vi "Report.vi"(6 "Printer Name":string, 8 "error in":errorcluster, 10 "Print/Preview":bool, 11 "Data In":T1) -> (0 "error out":errorcluster, 3 "Data Out":T1)   [LabVIEW 2025]
uses:
  <vilib>/Utility/NIReport.llb/NI_report.lvclass
  <vilib>/Utility/NIReport.llb/image depth.ctl
  <vilib>/Utility/NIReport.llb/NI_ReportGenerationCore.lvlib
  <vilib>/Utility/NIReport.llb/Report Type.ctl
  <vilib>/Utility/NIReport.llb/HTML Report Image Alignment.ctl
  <vilib>/Utility/NIReport.llb/Append Report Text (str wrap).vi
  <vilib>/printing/OpenHTMLReport.llb/Open HTML Report in Browser (Refnum).vi
  Controls/Tension_Output.ctl
  Controls/Nippel Turn Direction.ctl
  Controls/Runout Output.ctl
  Controls/Aditional Info.ctl
  Controls/Spork plot.ctl
  Controls/Spork type.ctl
  Controls/Spoke_stats.ctl
  Controls/Tension.ctl
  Controls/Runout.ctl
  Controls/Wheel_data.ctl
panel:
  out "Aditional Information":T10
  out "Spork Measured":i32[](array[numeric])
  out "Runout Measurement":T8[](array[typedef]) caption="Runout Value      Adjustment"
  out "Tencion Left":T6[](array[typedef]) caption="Tencion Left [kgf]    Pass?"
  out "Tencion Right":T6[](array[typedef]) caption="Tencion Right [kgf]   Pass?"
  out "Spokes Tension":cluster{dbl[], dbl[]}[](graph)
  out "Runout":T2[](graph)
  out "Wheel Visualation":cluster{dbl[], dbl[]}[](graph)
  # "Tension [kgf]"
  # "Pass?"
  # "Tension [kgf]"
  # "Pass?"
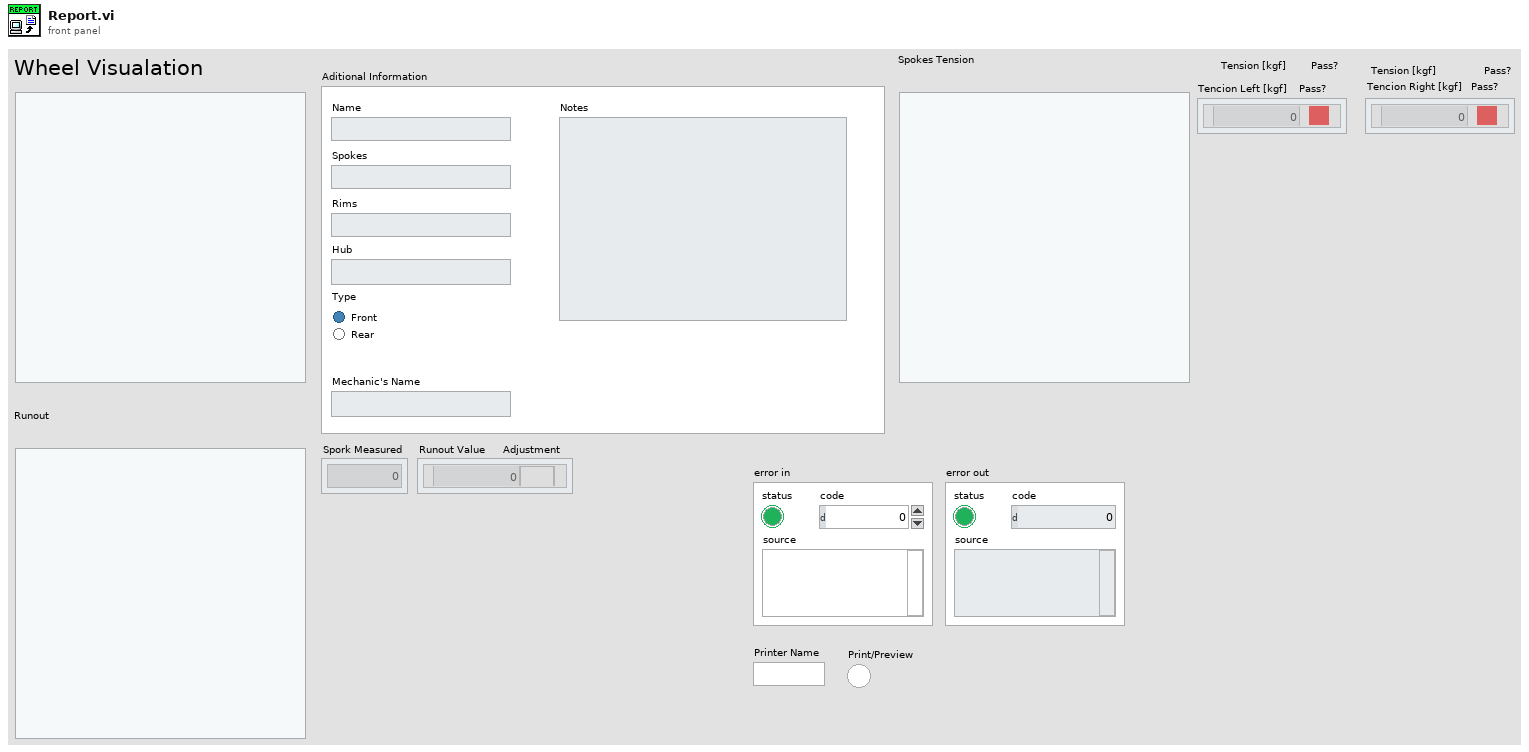
[diagram p1: front panel]
types:
  T1 = typedef "Wheel_data.ctl" = cluster{"Wheel Grapth":T2[], "Spokes":T3, "Tension":T5, "Runout":T7, "Avaliable Printers":string[], "Aditional Info":T10}
  T2 = typedef "Spork plot.ctl" = cluster{"X":dbl[], "Y":dbl[]}
  T3 = typedef "Spoke_stats.ctl" = cluster{"Spokes number":i32, "Spokes crosses":i32, "Spokes Type":T4}
  T4 = typedef "Spork type.ctl" = enum16{"Steel 1.4mm", "Steel 1.5mm", "Steel 1.6mm", "Steel 1.7mm", "Steel 1.8mm", "Steel 2mm", "Steel 2.3mm", "Steel 2.5mm", "Steel 2.6mm", "Aluminum 2.28mm", "Aluminum 2.54mm", "Aluminum 2.8mm", "Aluminum 3.3mm"}
  T5 = typedef "Tension.ctl" = cluster{"Spokes Tension Left":dbl[], "Tension Graph":T2[], "Average Left":dbl, "Variance":dbl, "Std Div Left":dbl, "Average Right":dbl, "Std Div Right":dbl, "Tension Output Left":T6[], "Tension Output Right":T6[], "Spokes Tension Right":dbl[]}
  T6 = typedef "Tension_Output.ctl" = cluster{"Tenction [kgf]":dbl, "Within Limit":bool}
  T7 = typedef "Runout.ctl" = cluster{"Runout Output":T8[], "Runout Graph":T2[], "Average":dbl, "Std Div":dbl, "Spoke Measured":i32[]}
  T8 = typedef "Runout Output.ctl" = cluster{"Value":dbl, "Nippel Direction":T9}
  T9 = typedef "Nippel Turn Direction.ctl" = u16
  T10 = typedef "Aditional Info.ctl" = cluster{"Name":string, "Rims":string, "Hub":string, "Notes":string, "Spokes":string, "Type":enum32{"Item 0", "Item 1"}, "Mechanic's Name":string}
  T11 = typedef "NI_ReportGenerationCore.lvlib/image depth.ctl" = u16
  T12 = typedef "NI_ReportGenerationCore.lvlib/HTML Report Image Alignment.ctl" = enum16{"(default)", "LEFT", "RIGHT", "TOP", "TEXTTOP", "MIDDLE", "ABSMIDDLE", "BASELINE", "BOTTOM", "ABSBOTTOM"}
  T13 = typedef "NI_ReportGenerationCore.lvlib/Report Type.ctl" = enum16{"HTML", "Word", "Excel"}
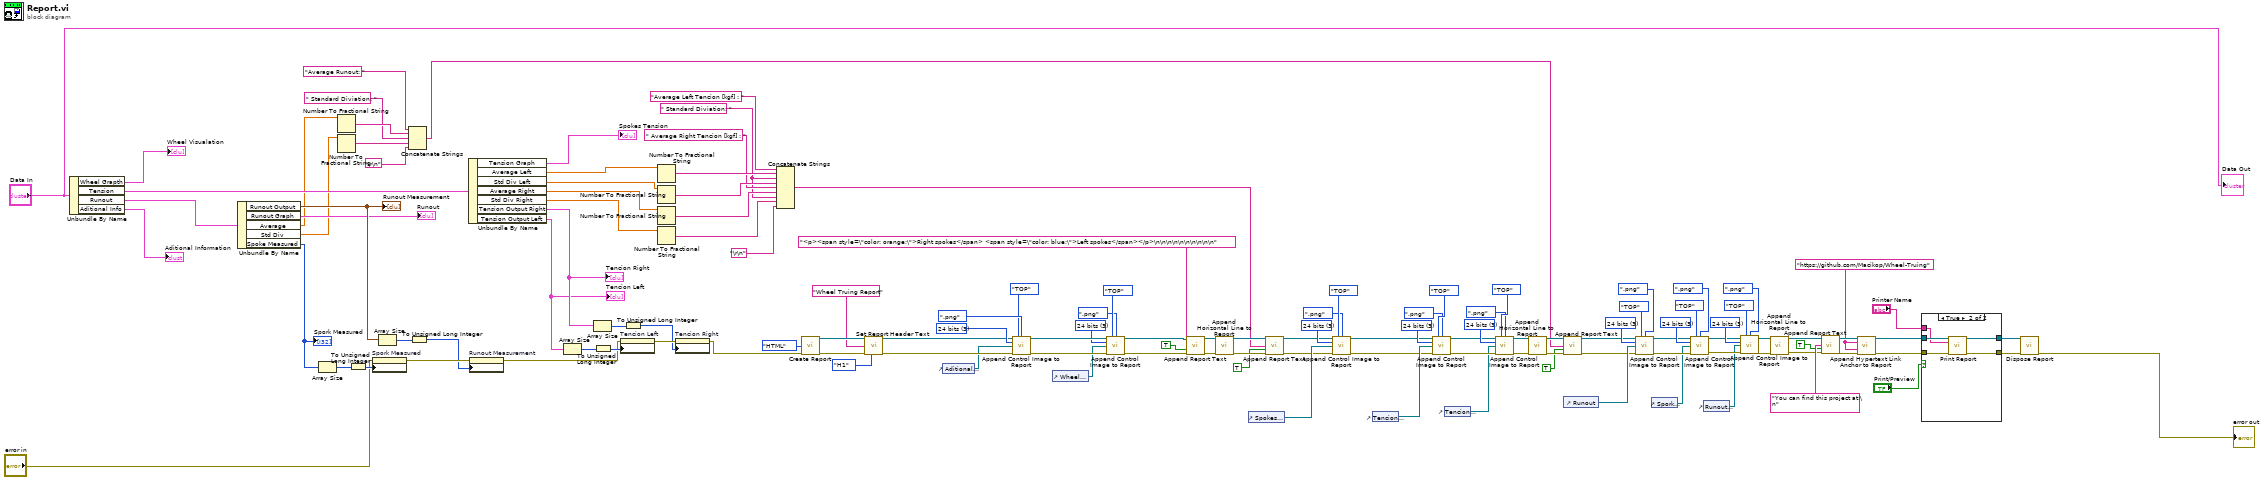
[diagram p0: block diagram]
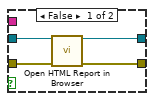
[diagram p2: hidden frame]
diagram:
  w35 = " Standard Diviation: " ("string")
  w66 = T11 3 items=["B&W", "4 bits", "8 bits", "24 bits"] ("image depth")
  w72 = T11 3 items=["B&W", "4 bits", "8 bits", "24 bits"] ("image depth")
  w76 = T11 3 items=["B&W", "4 bits", "8 bits", "24 bits"] ("image depth")
  w86 = T11 3 items=["B&W", "4 bits", "8 bits", "24 bits"] ("image depth")
  w92 = T11 3 items=["B&W", "4 bits", "8 bits", "24 bits"] ("image depth")
  w98 = T11 3 items=["B&W", "4 bits", "8 bits", "24 bits"] ("image depth")
  w103 = T11 3 items=["B&W", "4 bits", "8 bits", "24 bits"] ("image depth")
  w124 = T11 3 items=["B&W", "4 bits", "8 bits", "24 bits"] ("image depth")
  w108 = "https://github.com/Macikop/Wheel-Truing" ("URL of link - href")
  n1 = Unbundle By Name("Data In") -> ("Wheel Grapth"=→"Wheel Visualation":T2[], "Tension"=w51:T5, "Runout"=w27:T7, "Aditional Info"=→"Aditional Information":T10)
  n2 = Unbundle By Name(w27) -> ("Runout Output"=w24:T8[], "Runout Graph"=→"Runout":T2[], "Average"=w13:dbl, "Std Div"=w12:dbl, "Spoke Measured"=w22:i32[])
  "Runout Measurement" <- w24
  "Spork Measured" <- w22
  n3 = Array Size(array=w22) -> (size(s)=w28:i32)
  n4 = Number To Fractional String(number=w13) -> (F-format string=w11:string)  [unwired: 3 in]
  n5 = Number To Fractional String(number=w12) -> (F-format string=w10:string)  [unwired: 3 in]
  n6 = To Unsigned Long Integer(number=w28) -> (unsigned 32bit integer=w29:u32)
  n7 = property on="Spork Measured" class="Arr (strict)"(error in="error in", "Number of Rows"=w29) -> (error out=w32:errorcluster)  [unwired: 1 in, 1 out]
  n8 = Array Size(array=w24) -> (size(s)=w30:i32)
  n9 = Concatenate Strings("Average Runout: " ("string"), w11, " Standard Diviation: " ("string"), w10, "\r\n") -> (w7:string)
  n10 = To Unsigned Long Integer(number=w30) -> (unsigned 32bit integer=w31:u32)
  n11 = Unbundle By Name(w51) -> ("Tension Graph"=→"Spokes Tension":T2[], "Average Left"=w44:dbl, "Std Div Left"=w43:dbl, "Average Right"=w42:dbl, "Std Div Right"=w41:dbl, "Tension Output Right"=w26:T6[], "Tension Output Left"=w25:T6[])
  "Tencion Right" <- w26
  "Tencion Left" <- w25
  n12 = property on="Runout Measurement" class="Arr (strict)"(error in=w32, "Number of Rows"=w31) -> (error out=w21:errorcluster)  [unwired: 1 in, 1 out]
  n13 = Array Size(array=w25) -> (size(s)=w48:i32)
  n14 = Array Size(array=w26) -> (size(s)=w46:i32)
  n15 = To Unsigned Long Integer(number=w48) -> (unsigned 32bit integer=w49:u32)
  n16 = property on="Tencion Left" class="Arr (strict)"(error in=w21, "Number of Rows"=w49) -> (error out=w50:errorcluster)  [unwired: 1 in, 1 out]
  n17 = To Unsigned Long Integer(number=w46) -> (unsigned 32bit integer=w47:u32)
  n18 = Number To Fractional String(number=w44) -> (F-format string=w39:string)  [unwired: 3 in]
  n19 = Number To Fractional String(number=w43) -> (F-format string=w38:string)  [unwired: 3 in]
  n20 = Number To Fractional String(number=w42) -> (F-format string=w36:string)  [unwired: 3 in]
  n21 = Number To Fractional String(number=w41) -> (F-format string=w34:string)  [unwired: 3 in]
  n22 = property on="Tencion Right" class="Arr (strict)"(error in=w50, "Number of Rows"=w47) -> (error out=w20:errorcluster)  [unwired: 1 in, 1 out]
  n23 = Concatenate Strings("Average Left Tencion [kgf] : " ("string"), w39, w35, w38, " Average Right Tencion [kgf] : " ("string"), w36, w35, w34, "\r\n") -> (w33:string)
  n24 = call <vilib>:"Create Report.vi"("report type"=Report_Type."HTML" ("Report Type"), "error in (no error)"=w20) -> ("report out"=w127:refnum<class "NI_report.lvclass">, "error out"=w128:errorcluster)  [unwired: 12 in]
  n25 = call-dynamic "Set Report Header Text.vi"("report in"=w127, "center header text"="Wheel Truing Report", "error in (no error)"=w128, "HTML header size"=enum16{"H1", "H2", "H3", "H4", "H5", "H6", "H7"}."H1") -> ("report out"=w93:refnum<class "NI_report.lvclass">, "error out"=w94:errorcluster)  [unwired: 10 in]
  n26 = control-ref of="Aditional Information"() -> (w4:refnum<vi>)
  n27 = call-dynamic "Append Control Image to Report.vi"("report in"=w93, "alignment (default)"=HTML_Report_Image_Alignment."TOP", "image file type (.jpg)"=enum16{".jpg", ".png"}.".png" ("image file type"), "image depth"=w124, "ctrl reference"=w4, "error in (no error)"=w94) -> ("report out"=w104:refnum<class "NI_report.lvclass">, "error out"=w107:errorcluster)  [unwired: 6 in, 2 out]
  n28 = control-ref of="Wheel Visualation"() -> (w3:refnum<vi>)
  n29 = call-dynamic "Append Control Image to Report.vi"("report in"=w104, "alignment (default)"=HTML_Report_Image_Alignment."TOP", "image file type (.jpg)"=enum16{".jpg", ".png"}.".png", "image depth"=w103, "ctrl reference"=w3, "error in (no error)"=w107) -> ("report out"=w106:refnum<class "NI_report.lvclass">, "error out"=w105:errorcluster)  [unwired: 6 in, 2 out]
  n30 = call-poly <vilib>:"Append Report Text.vi"("report in"=w106, "text"="<p><span style=\"color: orange;\">Right spokes</span> <span style=\"color: blue;\">Left spokes</span></p>\n\n\n\n\n\n\n\n\n\n", "append on new line? (F)"=TRUE, "error in (no error)"=w105) -> ("report out"=w100:refnum<class "NI_report.lvclass">, "error out"=w99:errorcluster)  [unwired: 8 in, 2 out]
  n31 = call-dynamic "Append Horizontal Line to Report.vi"("report in"=w100, "error in (no error)"=w99) -> ("report out"=w58:refnum<class "NI_report.lvclass">, "error out"=w57:errorcluster)  [unwired: 12 in]
  n32 = control-ref of="Spokes Tension"() -> (w95:refnum<vi>)
  n33 = call-poly <vilib>:"Append Report Text.vi"("report in"=w58, "text"=w33, "append on new line? (F)"=TRUE, "error in (no error)"=w57) -> ("report out"=w55:refnum<class "NI_report.lvclass">, "error out"=w56:errorcluster)  [unwired: 8 in, 2 out]
  n34 = call-dynamic "Append Control Image to Report.vi"("report in"=w55, "alignment (default)"=HTML_Report_Image_Alignment."TOP", "image file type (.jpg)"=enum16{".jpg", ".png"}.".png", "image depth"=w98, "ctrl reference"=w95, "error in (no error)"=w56) -> ("report out"=w87:refnum<class "NI_report.lvclass">, "error out"=w88:errorcluster)  [unwired: 6 in, 2 out]
  n35 = control-ref of="Tencion Left"() -> (w89:refnum<vi>)
  n36 = call-dynamic "Append Control Image to Report.vi"("report in"=w87, "alignment (default)"=HTML_Report_Image_Alignment."TOP", "image file type (.jpg)"=enum16{".jpg", ".png"}.".png", "image depth"=w92, "ctrl reference"=w89, "error in (no error)"=w88) -> ("report out"=w82:refnum<class "NI_report.lvclass">, "error out"=w83:errorcluster)  [unwired: 6 in, 2 out]
  n37 = control-ref of="Tencion Right"() -> (w81:refnum<vi>)
  n38 = call-dynamic "Append Control Image to Report.vi"("report in"=w82, "alignment (default)"=HTML_Report_Image_Alignment."TOP", "image file type (.jpg)"=enum16{".jpg", ".png"}.".png", "image depth"=w86, "ctrl reference"=w81, "error in (no error)"=w83) -> ("report out"=w79:refnum<class "NI_report.lvclass">, "error out"=w80:errorcluster)  [unwired: 6 in, 2 out]
  n39 = call-dynamic "Append Horizontal Line to Report.vi"("report in"=w79, "error in (no error)"=w80) -> ("report out"=w18:refnum<class "NI_report.lvclass">, "error out"=w17:errorcluster)  [unwired: 12 in]
  n40 = call-poly <vilib>:"Append Report Text.vi"("report in"=w18, "text"=w7, "append on new line? (F)"=TRUE, "error in (no error)"=w17) -> ("report out"=w15:refnum<class "NI_report.lvclass">, "error out"=w16:errorcluster)  [unwired: 8 in, 2 out]
  n41 = control-ref of="Runout"() -> (w75:refnum<vi>)
  n42 = call-dynamic "Append Control Image to Report.vi"("report in"=w15, "alignment (default)"=HTML_Report_Image_Alignment."TOP", "image file type (.jpg)"=enum16{".jpg", ".png"}.".png", "image depth"=w76, "ctrl reference"=w75, "error in (no error)"=w16) -> ("report out"=w71:refnum<class "NI_report.lvclass">, "error out"=w70:errorcluster)  [unwired: 6 in, 2 out]
  n43 = control-ref of="Spork Measured"() -> (w69:refnum<vi>)
  n44 = call-dynamic "Append Control Image to Report.vi"("report in"=w71, "alignment (default)"=HTML_Report_Image_Alignment."TOP", "image file type (.jpg)"=enum16{".jpg", ".png"}.".png", "image depth"=w72, "ctrl reference"=w69, "error in (no error)"=w70) -> ("report out"=w65:refnum<class "NI_report.lvclass">, "error out"=w62:errorcluster)  [unwired: 6 in, 2 out]
  n45 = control-ref of="Runout Measurement"() -> (w61:refnum<vi>)
  n46 = call-dynamic "Append Control Image to Report.vi"("report in"=w65, "alignment (default)"=HTML_Report_Image_Alignment."TOP", "image file type (.jpg)"=enum16{".jpg", ".png"}.".png", "image depth"=w66, "ctrl reference"=w61, "error in (no error)"=w62) -> ("report out"=w64:refnum<class "NI_report.lvclass">, "error out"=w63:errorcluster)  [unwired: 6 in, 2 out]
  n47 = call-dynamic "Append Horizontal Line to Report.vi"("report in"=w64, "error in (no error)"=w63) -> ("report out"=w109:refnum<class "NI_report.lvclass">, "error out"=w110:errorcluster)  [unwired: 12 in]
  n48 = call-poly <vilib>:"Append Report Text.vi"("report in"=w109, "text"="You can find this project at:\n", "append on new line? (F)"=TRUE, "error in (no error)"=w110) -> ("report out"=w112:refnum<class "NI_report.lvclass">, "error out"=w111:errorcluster)  [unwired: 8 in, 2 out]
  n49 = call-dynamic "Append Hypertext Link Anchor to Report.vi"("report in"=w112, "URL of link - href"=w108, "link text"=w108, "error in (no error)"=w111) -> ("report out"=w119:refnum<class "NI_report.lvclass">, "error out"=w118:errorcluster)  [unwired: 8 in, 2 out]
  n50 = case shown="True" "Print/Preview" {
    tunnel: w119 -> [w132 w134]
    tunnel: w118 -> [w131 w137]
    tunnel: [w130 w136] -> w117
    tunnel: [w129 w135] -> w116
    tunnel: "Printer Name" -> [_ w133]
    frame False {
      n51 = call-poly <vilib>:"Open HTML Report in Browser.vi"("report in"=w132, "error in (no error)"=w131) -> ("report out"=w129:refnum<class "NI_report.lvclass">, "error out"=w130:errorcluster)  [unwired: 11 in, 1 out]
    }
    frame True {
      n52 = call-dynamic "Print Report.vi"("report in"=w134, "printer name (default)"=w133, "error in (no error)"=w137) -> ("report out"=w135:refnum<class "NI_report.lvclass">, "error out"=w136:errorcluster)  [unwired: 11 in]
    }
  }
  n53 = call-dynamic "Dispose Report.vi"("report in"=w116, "error in (no error)"=w117) -> ("error out"=→"error out":errorcluster)  [unwired: 13 in]
  "Data Out" <- "Data In"
